vi "Run.vi"() -> ()   [LabVIEW 2019]
uses:
  App/Generic Test Stand/Generic Test Stand.lvclass
  App/Generic Test Stand/Generic Test Stand.lvclass/Generic Test Stand.ctl
  App/TS Framework/TS Framework.lvlib
panel:
  in  "Cryo Sep":bool caption="Button"
  in  "DeepU":bool caption="Button"
  in  "LNG Boiling":bool caption="Button"
  in  "Water Tunnel":bool caption="Button"
  in  "Heat Flow":bool caption="Button"
  in  "HTS":bool caption="Button"
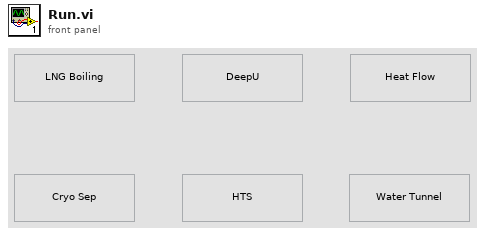
[diagram p1: front panel]
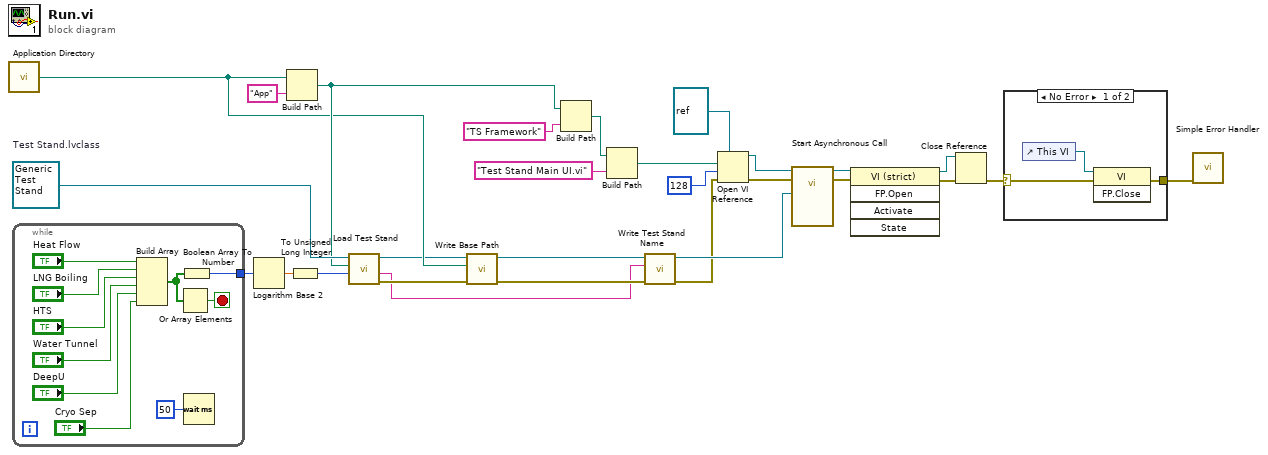
[diagram p0: block diagram]
diagram:
  w28 = refnum<class "Generic Test Stand.lvclass"> refnum  # Test Stand.lvclass
  n1 = call <vilib>:"Application Directory.vi"() -> ("Application Directory"=w25:path)
  n2 = while {
    tunnel: [w35] -> w24
    stop <- w37 stop-if-true
    n3 = Build Array("Heat Flow", "LNG Boiling", "HTS", "Water Tunnel", "DeepU", "Cryo Sep") -> (w36:bool[])
    n4 = Or Array Elements(Boolean array=w36) -> (logical OR=w37:bool)
    n5 = Boolean Array To Number(Boolean array=w36) -> (number=w35:u32)
    n6 = Wait (ms)(milliseconds to wait=u32 50) -> ()  [unwired: 1 out]
  }
  n7 = Logarithm Base 2(1:w24) -> (0:w23:dbl)
  n8 = Build Path(base path=w25, name or relative path="App") -> (appended path=w26:path)
  n9 = To Unsigned Long Integer(number=w23) -> (unsigned 32bit integer=w2:u32)
  n10 = call "Load Test Stand.vi"("Select Test Stand"=w2, "App Base Path"=w26, "Test Stand.lvclass"=w28) -> ("Error Out"=w6:errorcluster, "Test Stand Name"=w1:string, "Specific Test Stand.lvclass"=w9:refnum<class "Generic Test Stand.lvclass">)  [unwired: 6 in]
  n11 = call "Write Base Path.vi"("error in (no error)"=w6, "Base Path"=w25, "Generic Test Stand in"=w9) -> ("error out"=w5:errorcluster, "Generic Test Stand out"=w8:refnum<class "Generic Test Stand.lvclass">)  [unwired: 7 in]
  n12 = Build Path(base path=w26, name or relative path="TS Framework") -> (appended path=w10:path)
  n13 = Build Path(base path=w10, name or relative path="Test Stand Main UI.vi") -> (appended path=w17:path)
  n14 = call "Write Test Stand Name.vi"("error in (no error)"=w5, "Test Stand Name"=w1, "Generic Test Stand in"=w8) -> ("error out"=w4:errorcluster, "Generic Test Stand out"=w7:refnum<class "Generic Test Stand.lvclass">)  [unwired: 7 in]
  n15 = Open VI Reference(type specifier VI Refnum (for type only)=refnum<vi> refnum, vi path=w17, options=128, error in (no error)=w4) -> (vi reference=w19:refnum<vi>, error out=w18:errorcluster)  [unwired: 2 in]
  n16 = call-by-ref "Start Asynchronous Call"(reference=w19, error in=w18, "Test Stand.lvclass"=w7) -> (reference out=w16:refnum<vi>, error out=w14:errorcluster)  [unwired: 11 in]
  n17 = invoke class="VI (strict)" method="FP.Open"(reference=w16, error in=w14) -> (reference out=w15:refnum<vi>, error out=w13:errorcluster)  [unwired: 3 in, 3 out]
  n18 = Close Reference(reference=w15, error in (no error)=w13) -> (error out=w12:errorcluster)
  n19 = case shown="No Error" w12 {
    selector: w12 -> [w40 w42]
    tunnel: [w39 w42] -> w3
    frame No Error {
      n20 = control-ref of="This VI"() -> (w41:refnum<vi>)
      n21 = invoke class="VI" method="FP.Close"(reference=w41, error in=w40) -> (error out=w39:errorcluster)  [unwired: 1 in, 2 out]
    }
    frame Error {
    }
  }
  n22 = call <vilib>:"Simple Error Handler.vi"("error in (no error)"=w3) -> ()  [unwired: 4 in, 5 out]
